vi "WriteData.vi"(8 "error in":errorcluster, 11 "refnum in":refnum<file>) -> (0 "error out":errorcluster, 3 "refnum out":refnum<file>)   [LabVIEW 2016]
doc: "Logs data to csv file on roborio"
uses:
  Robot Global Data.vi
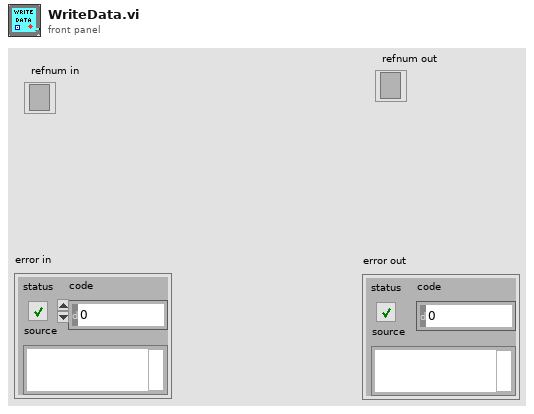
[diagram p1: front panel]
types:
  T1 = typedef "WPI_DriverStationRobotMode2.ctl" = enum16{"Autonomous Disabled", "Autonomous Enabled", "Teleop Disabled", "Teleop Enabled", "Disconnected", "Finish", "Test Disabled", "Test Enabled", "Emergency Stopped"}
  T2 = typedef "Z900_navX_Flags_OpStatusTypeDef.ctl" = u8
  T3 = typedef "Z900_navX_Flags_CalibrationStatusTypeDef.ctl" = u8
  T4 = cluster{"Update Rate Hz":u8, "Accelerometer Full-Scale Range":u8, "Gyro Full-Scale Range":u16, "OP Status":T2, "Calibration Status":T3, "Sensor Status":cluster{"MOVING":bool, "YAW_STABLE":bool, "MAG_DISTURBANCE":bool, "ALTITUDE_VALID":bool, "SEALEVEL_PRESS_SET":bool, "FUSED_HEADING_VALID":bool}, "Self Test Status":cluster{"Gyro Passed":bool, "Accel Passed":bool, "Mag Passed":bool, "Baro Passed":bool, "Complete":bool}}
  T5 = cluster{"Yaw":dbl, "Roll":dbl, "Pitch":dbl, "Heading":dbl, "Fused Heading":dbl}
  T6 = cluster{"LinearAcceleration X":dbl, "LinearAcceleration Y":dbl, "LinearAcceleration Z":dbl}
  T7 = cluster{"MOVING":bool, "YAW_STABLE":bool, "MAG_DISTURBANCE":bool, "ALTITUDE_VALID":bool, "SEALEVEL_PRESS_SET":bool, "FUSED_HEADING_VALID":bool}
  T8 = cluster{"Target?":bool, "Angle":dbl, "Distance":dbl, "NewAngle":dbl}
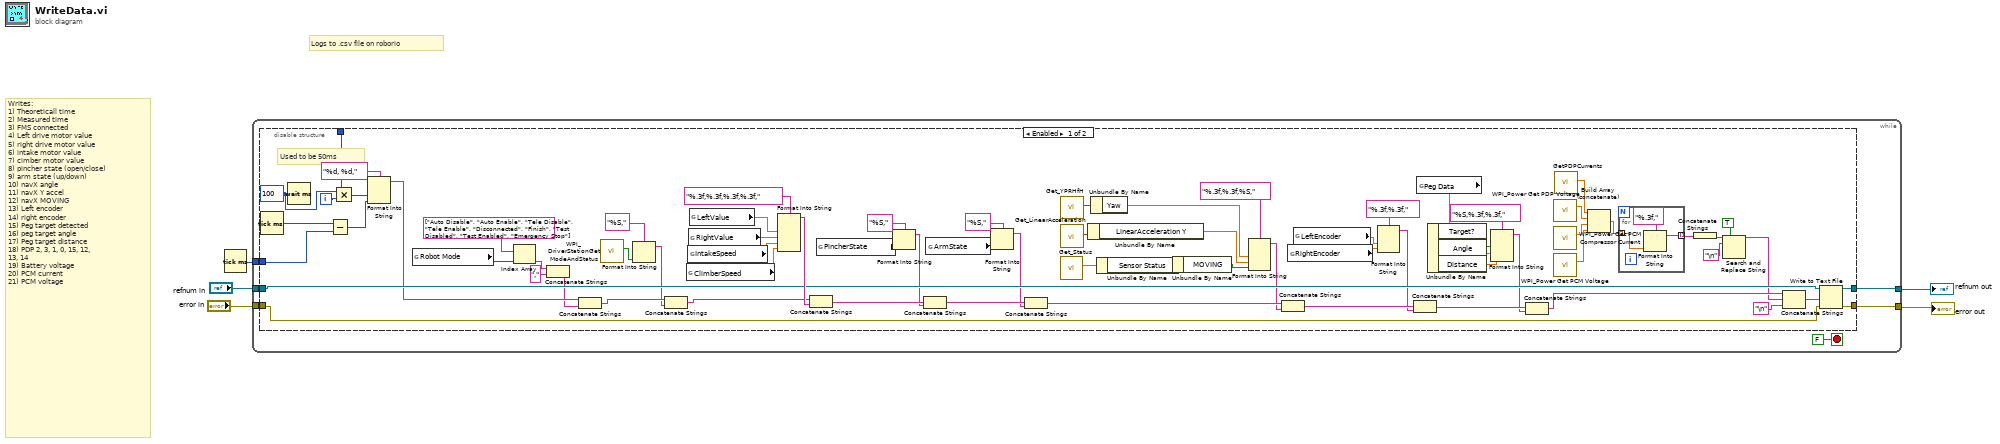
[diagram p0: block diagram]
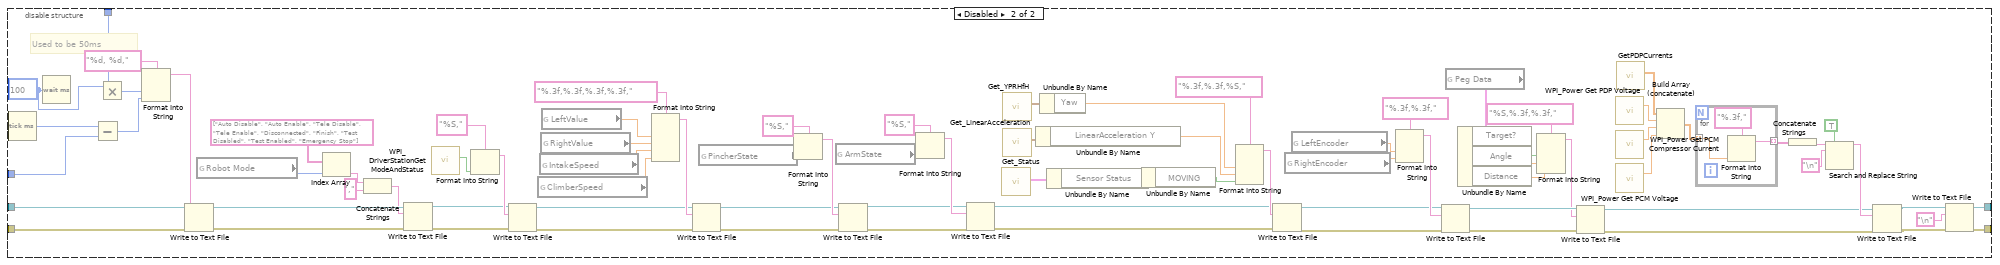
[diagram p2: hidden frame]
diagram:
  # "Logs to .csv file on roborio"
  # "Writes:\n1) Theoreticall time\n2) Measured time\n3) FMS connected\n4) Left drive motor value\n5) right drive motor value\n6) intake motor value\n7) cimber motor value\n8) pincher state (open/close)\n9) arm state (up/down)\n10) navX angle\n11) navX Y accel\n12) navX MOVING\n13) Left encoder\n14) right encoder\n15) Peg target detected\n16) peg target angle\n17) Peg target distance\n18) PDP 2, 3, 1, 0, 15, 12,\n13, 14\n19) Battery voltage\n20) PCM current\n21) PCM voltage"
  n1 = Tick Count (ms)() -> (millisecond timer value=w1:u32)
  n2 = while {
    tunnel: "error in" -> [w10]
    tunnel: "refnum in" -> [w9]
    tunnel: [w7] -> w3
    tunnel: [w8] -> w2
    tunnel: w1 -> [w6]
    i -> [w11]
    stop <- FALSE stop-if-true
    n3 = disable-structure shown="Enabled" {
      disable-tunnel: w11 -> [w82 w167]
      disable-tunnel: w10 -> [w30 w164]
      disable-tunnel: w9 -> [w31 w163]
      disable-tunnel: [w66 w141] -> w8
      disable-tunnel: [w65 w140] -> w7
      disable-tunnel: w6 -> [w37 w89]
      frame Enabled {
        w83 = u32 100 ("milliseconds to wait")
        # "Used to be 50ms"
        n4 = Tick Count (ms)() -> (millisecond timer value=w36:u32)
        n5 = Wait (ms)(milliseconds to wait=w83) -> ()  [unwired: 1 out]
        n6 = Subtract(x=w36, y=w37) -> (x-y=w35:u32)
        n7 = Multiply(x=w83, y=w82) -> (x*y=w81:u32)
        n8 = Format Into String(format string="%d, %d,", w81, w35) -> (resulting string=w29:string)  [unwired: 2 in, 1 out]
        n9 = global read "Robot Global Data.vi" "Robot Mode"() -> (w79:T1)
        n10 = Index Array(array=string[] ["Auto Disable", "Auto Enable", "Tele Disable", "Tele Enable", "Disconnected", "Finish", "Test Disabled", "Test Enabled", "Emergency Stop"], index=w79) -> (element=w57:string)
        n11 = Concatenate Strings(w57, "," ("string")) -> (w28:string)
        n12 = Concatenate Strings(w29, w28) -> (w27:string)
        n13 = call <vilib>:"WPI_DriverStationGetModeAndStatus.vi"() -> ("FMS Attached"=w53:bool)  [unwired: 10 in, 1 out]
        n14 = Format Into String(format string="%S,", w53) -> (resulting string=w26:string)  [unwired: 2 in, 1 out]
        n15 = Concatenate Strings(w27, w26) -> (w25:string)
        n16 = global read "Robot Global Data.vi" "ClimberSpeed"() -> (w47:dbl)
        n17 = global read "Robot Global Data.vi" "IntakeSpeed"() -> (w48:dbl)
        n18 = global read "Robot Global Data.vi" "RightValue"() -> (w76:dbl)
        n19 = global read "Robot Global Data.vi" "LeftValue"() -> (w77:dbl)
        n20 = Format Into String(format string="%.3f,%.3f,%.3f,%.3f,", w77, w76, w48, w47) -> (resulting string=w34:string)  [unwired: 2 in, 1 out]
        n21 = Concatenate Strings(w25, w34) -> (w24:string)
        n22 = global read "Robot Global Data.vi" "PincherState"() -> (w44:enum16{"Open", "Close"})
        n23 = Format Into String(format string="%S,", w44) -> (resulting string=w23:string)  [unwired: 2 in, 1 out]
        n24 = Concatenate Strings(w24, w23) -> (w22:string)
        n25 = global read "Robot Global Data.vi" "ArmState"() -> (w45:enum16{"Up", "Down"})
        n26 = Format Into String(format string="%S,", w45) -> (resulting string=w21:string)  [unwired: 2 in, 1 out]
        n27 = Concatenate Strings(w22, w21) -> (w20:string)
        n28 = call <vilib>:"Get_Status.vi"() -> ("Status"=w73:T4)  [unwired: 11 in]
        n29 = call <vilib>:"Get_YPRHfH.vi"() -> ("YRPHfH"=w50:T5)  [unwired: 11 in]
        n30 = call <vilib>:"Get_LinearAcceleration.vi"() -> ("Linear Acceleration"=w74:T6)  [unwired: 11 in]
        n31 = Unbundle By Name(w74) -> ("LinearAcceleration Y"=w71:dbl)
        n32 = Unbundle By Name(w50) -> ("Yaw"=w49:dbl)
        n33 = Unbundle By Name(w73) -> ("Sensor Status"=w72:T7)
        n34 = Unbundle By Name(w72) -> ("MOVING"=w70:bool)
        n35 = Format Into String(format string="%.3f,%.3f,%S,", w49, w71, w70) -> (resulting string=w19:string)  [unwired: 2 in, 1 out]
        n36 = Concatenate Strings(w20, w19) -> (w18:string)
        n37 = global read "Robot Global Data.vi" "RightEncoder"() -> (w59:dbl)
        n38 = global read "Robot Global Data.vi" "LeftEncoder"() -> (w58:dbl)
        n39 = Format Into String(format string="%.3f,%.3f,", w58, w59) -> (resulting string=w17:string)  [unwired: 2 in, 1 out]
        n40 = Concatenate Strings(w18, w17) -> (w16:string)
        n41 = global read "Robot Global Data.vi" "Peg Data"() -> (w42:T8)
        n42 = Unbundle By Name(w42) -> ("Target?"=w41:bool, "Angle"=w40:dbl, "Distance"=w39:dbl)
        n43 = Format Into String(format string="%S,%.3f,%.3f,", w41, w40, w39) -> (resulting string=w15:string)  [unwired: 2 in, 1 out]
        n44 = Concatenate Strings(w16, w15) -> (w14:string)
        n45 = call <vilib>:"WPI_Power Get PDP Voltage.vi"() -> ("voltage (V)"=w64:dbl)  [unwired: 14 in, 1 out]
        n46 = call <vilib>:"WPI_Power Get PCM Compressor Current.vi"() -> ("current (A)"=w55:dbl)  [unwired: 14 in, 1 out]
        n47 = call <vilib>:"WPI_Power Get PCM Voltage.vi"() -> ("Input Voltage"=w54:dbl)  [unwired: 13 in, 2 out]
        n48 = call "GetPDPCurrents.vi"() -> ("PDP Currents"=w51:dbl[])  [unwired: 11 in]
        n49 = Build Array (concatenate)(w51, w64, w55, w54) -> (w63:dbl[])
        n50 = for {
          tunnel: w63 -> [w86] mode=indexing
          tunnel: [w84] -> w62 mode=indexing
          n51 = Format Into String(format string="%.3f,", w86) -> (resulting string=w84:string)  [unwired: 2 in, 1 out]
        }
        n52 = Concatenate Strings(w62) -> (w61:string)
        n53 = Search and Replace String(replace all?=TRUE ("replace all? (F)"), input string=w61, search string="\n") -> (result string=w13:string)  [unwired: 5 in, 3 out]
        n54 = Concatenate Strings(w14, w13, "\n") -> (w33:string)
        n55 = Write to Text File(file (use dialog)=w31, text=w33, error in=w30) -> (refnum out=w65:refnum<file>, error out=w66:errorcluster)  [unwired: 1 in, 1 out]
      }
      frame Disabled {
        w168 = u32 100 ("milliseconds to wait")
        # "Used to be 50ms"
        n56 = Tick Count (ms)() -> (millisecond timer value=w88:u32)
        n57 = Wait (ms)(milliseconds to wait=w168) -> ()  [unwired: 1 out]
        n58 = Subtract(x=w88, y=w89) -> (x-y=w87:u32)
        n59 = Multiply(x=w168, y=w167) -> (x*y=w166:u32)
        n60 = Format Into String(format string="%d, %d,", w166, w87) -> (resulting string=w158:string)  [unwired: 2 in, 1 out]
        n61 = Write to Text File(file (use dialog)=w163, text=w158, error in=w164) -> (refnum out=w160:refnum<file>, error out=w159:errorcluster)  [unwired: 1 in, 1 out]
        n62 = global read "Robot Global Data.vi" "Robot Mode"() -> (w162:T1)
        n63 = Index Array(array=string[] ["Auto Disable", "Auto Enable", "Tele Disable", "Tele Enable", "Disconnected", "Finish", "Test Disabled", "Test Enabled", "Emergency Stop"], index=w162) -> (element=w130:string)
        n64 = Concatenate Strings(w130, "," ("string")) -> (w128:string)
        n65 = Write to Text File(file (use dialog)=w160, text=w128, error in=w159) -> (refnum out=w122:refnum<file>, error out=w121:errorcluster)  [unwired: 1 in, 1 out]
        n66 = call <vilib>:"WPI_DriverStationGetModeAndStatus.vi"() -> ("FMS Attached"=w125:bool)  [unwired: 10 in, 1 out]
        n67 = Format Into String(format string="%S,", w125) -> (resulting string=w123:string)  [unwired: 2 in, 1 out]
        n68 = Write to Text File(file (use dialog)=w122, text=w123, error in=w121) -> (refnum out=w120:refnum<file>, error out=w119:errorcluster)  [unwired: 1 in, 1 out]
        n69 = global read "Robot Global Data.vi" "ClimberSpeed"() -> (w114:dbl)
        n70 = global read "Robot Global Data.vi" "IntakeSpeed"() -> (w115:dbl)
        n71 = global read "Robot Global Data.vi" "RightValue"() -> (w156:dbl)
        n72 = global read "Robot Global Data.vi" "LeftValue"() -> (w157:dbl)
        n73 = Format Into String(format string="%.3f,%.3f,%.3f,%.3f,", w157, w156, w115, w114) -> (resulting string=w155:string)  [unwired: 2 in, 1 out]
        n74 = Write to Text File(file (use dialog)=w120, text=w155, error in=w119) -> (refnum out=w105:refnum<file>, error out=w104:errorcluster)  [unwired: 1 in, 1 out]
        n75 = global read "Robot Global Data.vi" "PincherState"() -> (w107:enum16{"Open", "Close"})
        n76 = Format Into String(format string="%S,", w107) -> (resulting string=w113:string)  [unwired: 2 in, 1 out]
        n77 = global read "Robot Global Data.vi" "ArmState"() -> (w108:enum16{"Up", "Down"})
        n78 = Write to Text File(file (use dialog)=w105, text=w113, error in=w104) -> (refnum out=w111:refnum<file>, error out=w110:errorcluster)  [unwired: 1 in, 1 out]
        n79 = Format Into String(format string="%S,", w108) -> (resulting string=w112:string)  [unwired: 2 in, 1 out]
        n80 = Write to Text File(file (use dialog)=w111, text=w112, error in=w110) -> (refnum out=w103:refnum<file>, error out=w102:errorcluster)  [unwired: 1 in, 1 out]
        n81 = call <vilib>:"Get_Status.vi"() -> ("Status"=w152:T4)  [unwired: 11 in]
        n82 = call <vilib>:"Get_YPRHfH.vi"() -> ("YRPHfH"=w117:T5)  [unwired: 11 in]
        n83 = call <vilib>:"Get_LinearAcceleration.vi"() -> ("Linear Acceleration"=w153:T6)  [unwired: 11 in]
        n84 = Unbundle By Name(w153) -> ("LinearAcceleration Y"=w150:dbl)
        n85 = Unbundle By Name(w117) -> ("Yaw"=w116:dbl)
        n86 = Unbundle By Name(w152) -> ("Sensor Status"=w151:T7)
        n87 = Unbundle By Name(w151) -> ("MOVING"=w149:bool)
        n88 = Format Into String(format string="%.3f,%.3f,%S,", w116, w150, w149) -> (resulting string=w147:string)  [unwired: 2 in, 1 out]
        n89 = Write to Text File(file (use dialog)=w103, text=w147, error in=w102) -> (refnum out=w145:refnum<file>, error out=w144:errorcluster)  [unwired: 1 in, 1 out]
        n90 = global read "Robot Global Data.vi" "RightEncoder"() -> (w132:dbl)
        n91 = global read "Robot Global Data.vi" "LeftEncoder"() -> (w131:dbl)
        n92 = Format Into String(format string="%.3f,%.3f,", w131, w132) -> (resulting string=w146:string)  [unwired: 2 in, 1 out]
        n93 = Write to Text File(file (use dialog)=w145, text=w146, error in=w144) -> (refnum out=w99:refnum<file>, error out=w98:errorcluster)  [unwired: 1 in, 1 out]
        n94 = global read "Robot Global Data.vi" "Peg Data"() -> (w97:T8)
        n95 = Unbundle By Name(w97) -> ("Target?"=w96:bool, "Angle"=w95:dbl, "Distance"=w94:dbl)
        n96 = Format Into String(format string="%S,%.3f,%.3f,", w96, w95, w94) -> (resulting string=w92:string)  [unwired: 2 in, 1 out]
        n97 = Write to Text File(file (use dialog)=w99, text=w92, error in=w98) -> (refnum out=w91:refnum<file>, error out=w90:errorcluster)  [unwired: 1 in, 1 out]
        n98 = call <vilib>:"WPI_Power Get PDP Voltage.vi"() -> ("voltage (V)"=w138:dbl)  [unwired: 14 in, 1 out]
        n99 = call <vilib>:"WPI_Power Get PCM Compressor Current.vi"() -> ("current (A)"=w127:dbl)  [unwired: 14 in, 1 out]
        n100 = call <vilib>:"WPI_Power Get PCM Voltage.vi"() -> ("Input Voltage"=w126:dbl)  [unwired: 13 in, 2 out]
        n101 = call "GetPDPCurrents.vi"() -> ("PDP Currents"=w118:dbl[])  [unwired: 11 in]
        n102 = Build Array (concatenate)(w118, w138, w127, w126) -> (w137:dbl[])
        n103 = for {
          tunnel: w137 -> [w171] mode=indexing
          tunnel: [w169] -> w136 mode=indexing
          n104 = Format Into String(format string="%.3f,", w171) -> (resulting string=w169:string)  [unwired: 2 in, 1 out]
        }
        n105 = Concatenate Strings(w136) -> (w135:string)
        n106 = Search and Replace String(replace all?=TRUE ("replace all? (F)"), input string=w135, search string="\n") -> (result string=w134:string)  [unwired: 5 in, 3 out]
        n107 = Write to Text File(file (use dialog)=w91, text=w134, error in=w90) -> (refnum out=w101:refnum<file>, error out=w100:errorcluster)  [unwired: 1 in, 1 out]
        n108 = Write to Text File(file (use dialog)=w101, text="\n", error in=w100) -> (refnum out=w140:refnum<file>, error out=w141:errorcluster)  [unwired: 1 in, 1 out]
      }
    }
  }
  "refnum out" <- w3
  "error out" <- w2
